vi "Read SuBus Script and Create HWS File .vi"() -> ()   [LabVIEW 2013]
uses:
  <vilib>/Utility/file.llb/Read From Spreadsheet File (string).vi
  <vilib>/Waveform/DWDTOps.llb/DWDT Boolean Array to Digital.vi
panel:
  out "name":string
  out "Digital Waveform Graph":digitalwaveform(graph)={"t0"=timestamp(0 s since 1904-01-01), "dt"=5e-08, "Y"={"transitions"=[], "data"=[[0], [0], [0], [0], [0], [0], [0], [0], [1], [1], [1], [1], [1], [1], [1], [1], [1], [1], [1], [1], [1], [1], [1], [1], [1], [1], [1], [1], [1], [1], [1], [1], [1], [1], [1], [1], [1], [1], [1], [1], [0], [0], [0], [0], [0], [0], [0], [0], [0], [0], [0], [0], [1], [1], [1], [1], [0], [0], [0], [0], [1], [1], [1], [1], [1], [1], [1], [1], [1], [1], [1], [1], [0], [0], [0], [0], [0], [0], [0], [0], [0], [0], [0], [0], [1], [1], [1], [1], [0], [0], [0], [0], [0], [0], [0], [0], [0], [0], [0], [0], [1], [1], [1], [1], [0], [0], [0], [0], [1], [1], [1], [1], [1], [1], [1], [1], [1], [1], [1], [1], [0], [0], [0], [0], [0], [0], [0], [0], [0], [0], [0], [0], [1], [1], [1], [1], [0], [0], [0], [0], [0], [0], [0], [0], [0], [0], [0], [0], [1], [1], [1], [1], [0], [0], [0], [0], [1], [1], [1], [1], [1], [1], [1], [1], [1], [1], [1], [1], [0], [0], [0], [0], [1], [1], [1], [1], [1], [1], [1], [1], [1], [1], [1], [1], [0], [0], [0], [0], [1], [1], [1], [1], [1], [1], [1], [1], [1], [1], [1], [1], [0], [0], [0], [0], [1], [1], [1], [1], [1], [1], [1], [1], [1], [1], [1], [1], [0], [0], [0], [0], [1], [1], [1], [1], [1], [1], [1], [1], [1], [1], [1], [1], [0], [0], [0], [0], [0], [0], [0], [0], [0], [0], [0], [0], [1], [1], [1], [1], [0], [0], [0], [0], [0], [0], [0], [0], [0], [0], [0], [0], [1], [1], [1], [1], [0], [0], [0], [0], [0], [0], [0], [0], [0], [0], [0], [0], [1], [1], [1], [1], [0], [0], [0], [0], [1], [1], [1], [1], [1], [1], [1], [1], [1], [1], [1], [1], [0], [0], [0], [0], [0], [0], [0], [0], [0], [0], [0], [0], [1], [1], [1], [1], [0], [0], [0], [0], [0], [0], [0], [0], [0], [0], [0], [0], [1], [1], [1], [1], [0], [0], [0], [0], [0], [0], [0], [0], [0], [0], [0], [0], [1], [1], [1], [1], [0], [0], [0], [0], [1], [1], [1], [1], [1], [1], [1], [1], [1], [1], [1], [1], [0], [0], [0], [0], [0], [0], [0], [0], [0], [0], [0], [0], [1], [1], [1], [1], [0], [0], [0], [0], [0], [0], [0], [0], [0], [0], [0], [0], [1], [1], [1], [1], [0], [0], [0], [0], [0], [0], [0], [0], [0], [0], [0], [0], [1], [1], [1], [1], [0], [0], [0], [0], [0], [0], [0], [0], [0], [0], [0], [0], [1], [1], [1], [1], [0], [0], [0], [0], [0], [0], [0], [0], [0], [0], [0], [0], [1], [1], [1], [1], [0], [0], [0], [0], [0], [0], [0], [0], [0], [0], [0], [0], [1], [1], [1], [1], [0], [0], [0], [0], [0], [0], [0], [0], [0], [0], [0], [0], [1], [1], [1], [1], [0], [0], [0], [0], [1], [1], [1], [1], [1], [1], [1], [1], [1], [1], [1], [1], [0], [0], [0], [0], [1], [1], [1], [1], [1], [1], [1], [1], [1], [1], [1], [1], [0], [0], [0], [0], [1], [1], [1], [1], [1], [1], [1], [1], [1], [1], [1], [1], [0], [0], [0], [0], [0], [0], [0], [0], [0], [0], [0], [0], [1], [1], [1], [1], [0], [0], [0], [0], [0], [0], [0], [0], [0], [0], [0], [0], [1], [1], [1], [1], [0], [0], [0], [0], [1], [1], [1], [1], [1], [1], [1], [1], [1], [1], [1], [1], [0], [0], [0], [0], [0], [0], [0], [0], [0], [0], [0], [0], [0], [0], [0], [0]]}}
  out "Array":string[](array[string])=["@ REPV 8 0", "@ REPV 20 1", "@ REPV C 0", "@ REPV 4 1", "@ REPV 4 0", "@ REPV C 1", "@ REPV C 0", "@ REPV 4 1", "@ REPV C 0", "@ REPV 4 1", "@ REPV 4 0", "@ REPV C 1", "@ REPV C 0", "@ REPV 4 1", "@ REPV C 0", "@ REPV 4 1", "@ REPV 4 0", "@ REPV C 1", "@ REPV 4 0", "@ REPV C 1", "@ REPV 4 0", "@ REPV C 1", "@ REPV 4 0", "@ REPV C 1", "@ REPV 4 0", "@ REPV C 1", "@ REPV C 0", "@ REPV 4 1", "@ REPV C 0", "@ REPV 4 1", "@ REPV C 0", "@ REPV 4 1", "@ REPV 4 0", "@ REPV C 1", "@ REPV C 0", "@ REPV 4 1", "@ REPV C 0", "@ REPV 4 1", "@ REPV C 0", "@ REPV 4 1", "@ REPV 4 0", "@ REPV C 1", "@ REPV C 0", "@ REPV 4 1", "@ REPV C 0", "@ REPV 4 1", "@ REPV C 0", "@ REPV 4 1", "@ REPV C 0", "@ REPV 4 1", "@ REPV C 0", "@ REPV 4 1", "@ REPV C 0", "@ REPV 4 1", "@ REPV C 0", "@ REPV 4 1", "@ REPV 4 0", "@ REPV C 1", "@ REPV 4 0", "@ REPV C 1", "@ REPV 4 0", "@ REPV C 1", "@ REPV C 0", "@ REPV 4 1", "@ REPV C 0", "@ REPV 4 1", "@ REPV 4 0", "@ REPV C 1", "@ REPV 4 L", "@ REPV 4 H", "@ REPV 8 H"]
  out "all rows":string[][](array[string])=[[""], ["; ************** Slave SuBus Write **************"], ["; **** Generate SuBus Training Sequence 50%Lo, 200%Hi, 75%Lo, 25%Hi, 25%Lo, 75%Hi ****"], ["@ REPV 8 0"], ["@ REPV 20 1"], ["@ REPV C 0"], ["@ REPV 4 1"], ["@ REPV 4 0"], ["@ REPV C 1"], ["; **** Generate SuBus Command & Data Frame ****"], ["@ REPV C 0"], ["@ REPV 4 1"], ["@ REPV C 0"], ["@ REPV 4 1"], ["@ REPV 4 0"], ["@ REPV C 1"], ["@ REPV C 0"], ["@ REPV 4 1"], ["@ REPV C 0"], ["@ REPV 4 1"], ["@ REPV 4 0"], ["@ REPV C 1"], ["@ REPV 4 0"], ["@ REPV C 1"], ["@ REPV 4 0"], ["@ REPV C 1"], ["@ REPV 4 0"], ["@ REPV C 1"], ["@ REPV 4 0"], ["@ REPV C 1"], ["@ REPV C 0"], ["@ REPV 4 1"], ["@ REPV C 0"], ["@ REPV 4 1"], ["@ REPV C 0"], ["@ REPV 4 1"], ["@ REPV 4 0"], ["@ REPV C 1"], ["@ REPV C 0"], ["@ REPV 4 1"], ["@ REPV C 0"], ["@ REPV 4 1"], ["@ REPV C 0"], ["@ REPV 4 1"], ["@ REPV 4 0"], ["@ REPV C 1"], ["@ REPV C 0"], ["@ REPV 4 1"], ["@ REPV C 0"], ["@ REPV 4 1"], ["@ REPV C 0"], ["@ REPV 4 1"], ["@ REPV C 0"], ["@ REPV 4 1"], ["@ REPV C 0"], ["@ REPV 4 1"], ["@ REPV C 0"], ["@ REPV 4 1"], ["@ REPV C 0"], ["@ REPV 4 1"], ["@ REPV 4 0"], ["@ REPV C 1"], ["@ REPV 4 0"], ["@ REPV C 1"], ["@ REPV 4 0"], ["@ REPV C 1"], ["@ REPV C 0"], ["@ REPV 4 1"], ["@ REPV C 0"], ["@ REPV 4 1"], ["@ REPV 4 0"], ["@ REPV C 1"], ["; **** Compare For ACK/NACK ****"], ["@ REPV 4 L"], ["@ REPV 4 H"], ["@ REPV 8 H"], [";"], [""], [""]]
  in  "file path (dialog if empty)":path=path "C:/Users/er080167/Documents/XP2100/Prototypes/SuBUS/RffeSuBusScriptFile_0x1c_D128.txt"
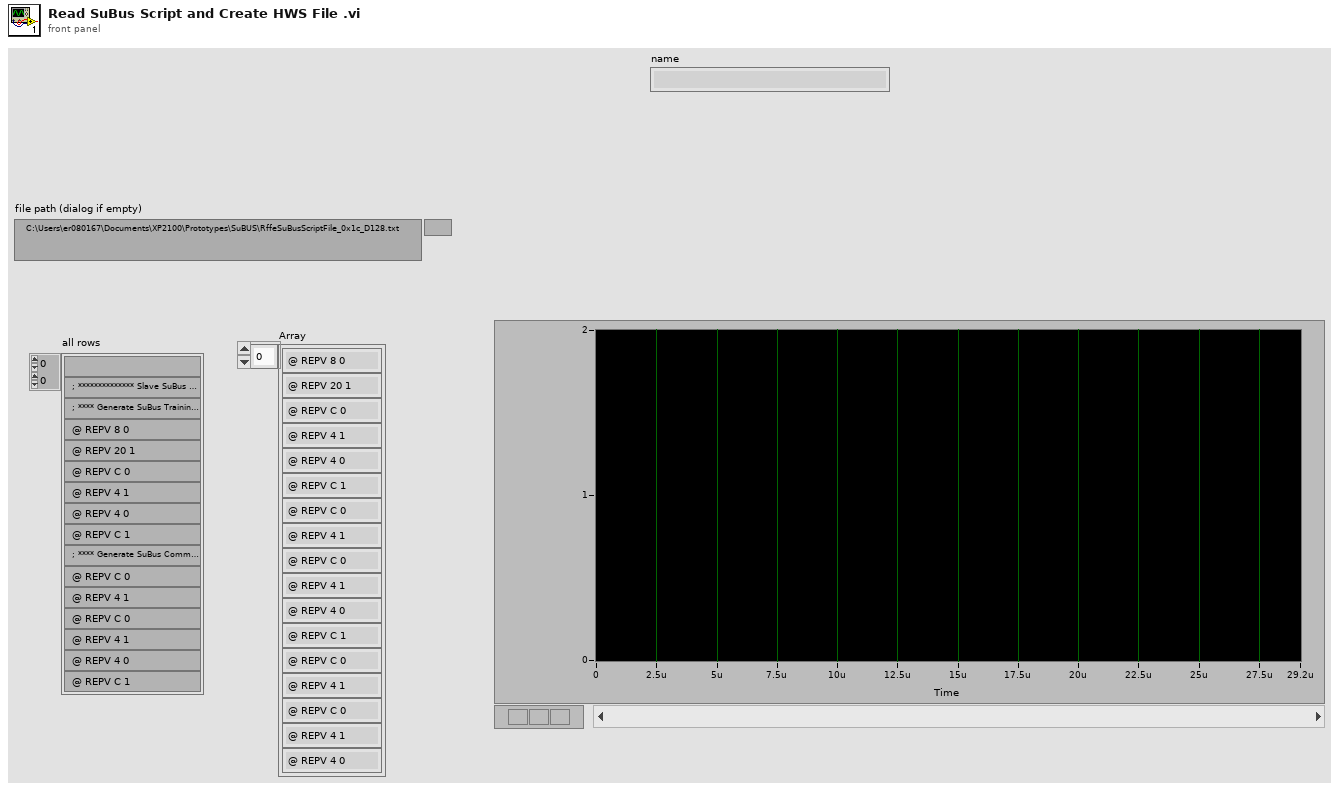
[diagram p1: front panel]
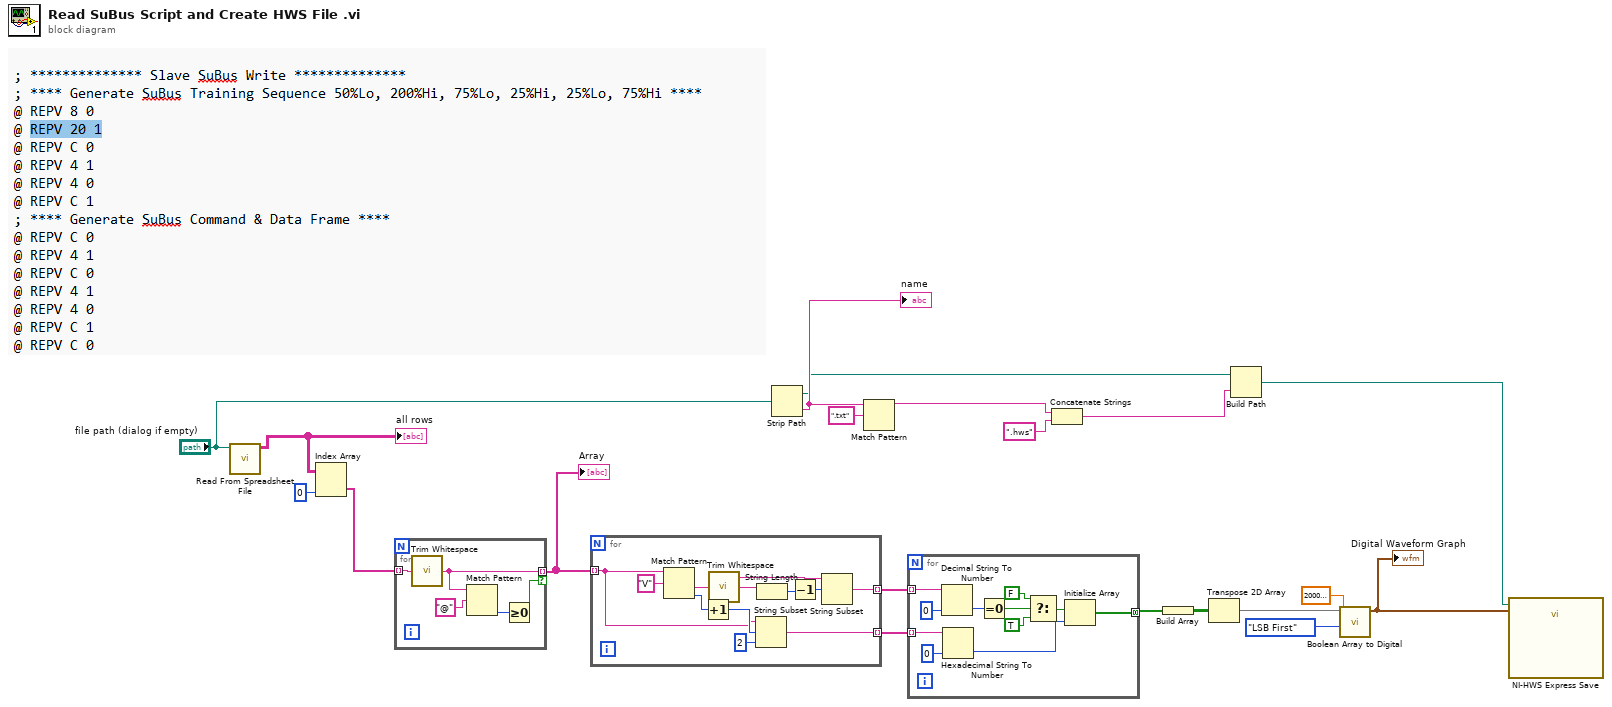
[diagram p0: block diagram]
diagram:
  n1 = call-poly <vilib>:"Read From Spreadsheet File.vi"("file path (dialog if empty)"="file path (dialog if empty)") -> ("all rows"=w20:string[][])  [unwired: 6 in, 4 out]
  "all rows" <- w20
  n2 = Index Array(array=w20, index (col)=0 ("disabled index (col)")) -> (element=w18:string[])  [unwired: 1 in]
  n3 = for {
    tunnel: w18 -> [w25] mode=indexing
    tunnel: [w23] -> w17 mode=indexing if=w21
    n4 = call <vilib>:"Trim Whitespace.vi"("string"=w25) -> ("trimmed string"=w23:string)  [unwired: 1 in]
    n5 = Match Pattern(string=w23, regular expression="@") -> (offset past match=w22:i32)  [unwired: 1 in, 3 out]
    n6 = Greater Or Equal To 0?(x=w22) -> (x >= 0?=w21:bool)
  }
  "Array" <- w17
  n7 = for {
    tunnel: w17 -> [w26] mode=indexing
    tunnel: [w32] -> w16 mode=indexing
    tunnel: [w27] -> w15 mode=indexing
    n8 = Match Pattern(string=w26, regular expression="V") -> (after substring=w35:string, offset past match=w31:i32)  [unwired: 1 in, 2 out]
    n9 = Increment(x=w31) -> (x+1=w30:i32)
    n10 = call <vilib>:"Trim Whitespace.vi"("string"=w35) -> ("trimmed string"=w29:string)  [unwired: 1 in]
    n11 = String Subset(string=w26, offset (0)=w30, length (rest)=2 ("length (rest)")) -> (substring=w27:string)
    n12 = String Length(string=w29) -> (length=w34:i32)
    n13 = Decrement(x=w34) -> (x-1=w33:i32)
    n14 = String Subset(string=w29, offset (0)=w33) -> (substring=w32:string)  [unwired: 1 in]
  }
  n15 = Strip Path(path="file path (dialog if empty)") -> (stripped path=w2:path, name=w7:string)
  "name" <- w7
  n16 = Match Pattern(string=w7, regular expression=".txt") -> (before substring=w5:string)  [unwired: 1 in, 3 out]
  n17 = for {
    tunnel: w16 -> [w47] mode=indexing
    tunnel: w15 -> [w45] mode=indexing
    tunnel: [w37] -> w12 mode=concatenating
    n18 = Decimal String To Number(string=w47, default (0L)=i8 0 ("default (0 I32)")) -> (number=w43:i8)  [unwired: 1 in, 1 out]
    n19 = Hexadecimal String To Number(string=w45, default (0uL)=i8 0 ("default (0 I32)")) -> (number=w38:i8)  [unwired: 1 in, 1 out]
    n20 = Equal To 0?(x=w43) -> (x = 0?=w42:bool)
    n21 = Select(t=FALSE, s=w42, f=TRUE) -> (s? t:f=w39:bool)
    n22 = Initialize Array(w39, w38) -> (w37:bool[])
  }
  n23 = Concatenate Strings(w5, ".hws" ("regular expression")) -> (w3:string)
  n24 = Build Array(w12) -> (w11:bool[][])
  n25 = Transpose 2D Array(2D array=w11) -> (transposed array=w10:bool[][])
  n26 = Build Path(base path=w2, name or relative path=w3) -> (appended path=w1:path)
  n27 = call-poly <vilib>:"Boolean Array to Digital.vi"("mode"=enum16{"LSB First", "MSB First"}."LSB First", "sample rate"=20000000.0, "boolean array"=w10) -> ("digital waveform"=w9:digitalwaveform)  [unwired: 7 in, 1 out]
  "Digital Waveform Graph" <- w9
  n28 = call "NI-HWS Express Save"("digital waveform"=w9, "file path"=w1) -> ()  [unwired: 9 in, 1 out]
